vi "Filter_array.vi"(7 "order":i32=4, 10 "sampling freq: fs":dbl=1.0 format="%0.2f", 11 "Input":dbl[](array[numeric])) -> (3 "Filtered":dbl[](array[numeric]))   [LabVIEW 2016]
uses:
  <vilib>/Analysis/3filter.llb/Filter Passband Type.ctl
  <vilib>/Analysis/3filter.llb/Butterworth Filter (DBL).vi
  <vilib>/Analysis/NI_AALBase.lvlib
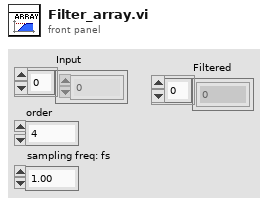
[diagram p1: front panel]
types:
  T1 = typedef "NI_AALBase.lvlib/Filter Passband Type.ctl" = enum32{"Lowpass", "Highpass", "Bandpass", "Bandstop"}
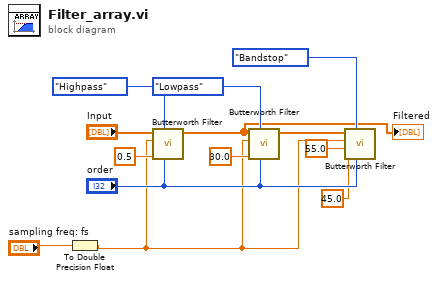
[diagram p0: block diagram]
diagram:
  n1 = To Double Precision Float(number="sampling freq: fs") -> (double precision float=w4:dbl)
  n2 = call-poly <vilib>:"Butterworth Filter.vi"("order"="order", "filter type"=Filter_Passband_Type."Highpass", "low cutoff freq: fl"=0.5, "sampling freq: fs"=w4, "X"="Input") -> ("Filtered X"=w1:dbl[])  [unwired: 3 in, 1 out]
  "Filtered" <- w1
  n3 = call-poly <vilib>:"Butterworth Filter.vi"("order"="order", "filter type"=Filter_Passband_Type."Lowpass", "low cutoff freq: fl"=30.0, "sampling freq: fs"=w4, "X"=w1) -> ("Filtered X"=w5:dbl[])  [unwired: 3 in, 1 out]
  n4 = call-poly <vilib>:"Butterworth Filter.vi"("order"="order", "filter type"=Filter_Passband_Type."Bandstop", "low cutoff freq: fl"=45.0, "high cutoff freq: fh"=55.0, "sampling freq: fs"=w4, "X"=w5) -> ()  [unwired: 2 in, 2 out]
